vi "Ecal-Manual-2.vi"(0 "PNA_IN":refnum<visa-resource-name>="TCPIP0::169.254.70.180::inst0::INSTR", 1 "RF_Switch_In":refnum<visa-resource-name>="GPIB0::29::INSTR", 5 "error in":errorcluster, 7 "Channel":i32=1, 8 "RecallFile":string="D:\\State Files\\WAM_PRODUCTION.csa", 9 "Save to File(t)":bool=TRUE, 11 "ByPassRfSwitch(t)":bool) -> (12 "Success?(t)":bool, 14 "VISA Out":refnum<visa-resource-name>="TCPIP0::169.254.70.180::inst0::INSTR", 15 "rfsw_out":refnum<visa-resource-name>, 19 "error out":errorcluster)   [LabVIEW 2018]
doc: "This VBScript program performs a Guided Calibration using Mechanical standards. While this example is good to use as a starting point for guided mechanical cal, the Guided comprehensive cal example has some advanced features that are not in this program.\n\nThe SCPI commands in this example are sent over a COM interface using the SCPIStringParser object. You do NOT need a GPIB connection to run this example.\n\nThis VBScript (*.vbs) program can be run as a macro in the PNA. To do this, copy the following code into a text editor file such as Notepad and save it on the PNA hard drive as Guided.vbs. Learn how to setup and run the macro.\n\n' Performing a 2-port cal (Ports 1 and 2)\n\nDim app\nDim scpi\n\n' Create / Get the PNA application.\nSet app = CreateObject(\"AgilentPNA835x.Application\")\nSet scpi = app.ScpiStringParser\n\n' Specify the DUT connectors\nscpi.Execute \"sens:corr:coll:guid:conn:port1 \"\"APC 3.5 female\"\" \"\nscpi.Execute \"sens:corr:coll:guid:conn:port2 \"\"APC 3.5 male\"\" \"\n\n' Note: If your PNA has more than 2 ports, you would need to uncomment\n' one or both of these next two lines, to explicitly specify this is\n' just a 2-port cal.\n'scpi.Execute \"sens:corr:coll:guid:conn:port3 \"\"Not used\"\" \"\n'scpi.Execute \"sens:corr:coll:guid:conn:port4 \"\"Not used\"\" \"\nMsgBox \"Connectors defined for Ports 1 and 2\" \n\n' Select the Cal Kit for each port being calibrated.\nscpi.Execute \"sens:corr:coll:guid:ckit:port1 \"\"85052D\"\" \"\nscpi.Execute \"sens:corr:coll:guid:ckit:port2 \"\"85052D\"\" \"\nMsgBox \"Cal kits defined for Ports 1 and 2\"\n\n' Initiate the calibration and query the number of steps\nscpi.Execute \"sens:corr:coll:guid:init\"\nnumSteps = scpi.Execute(\"sens:corr:coll:guid:steps?\")\nMsgBox \"Number of steps is \" + CStr(numSteps)\n\n' Measure the standards\n'The following series of commands shows that standards \n'can be measured in any order. These steps acquire \n'measurement of standards in reverse order.\n'It is easiest to iterate through standards using \n'a For-Next Loop.\nFor i = numSteps To 1\nstep = \"Step \" + CStr(i) + \" of \" + CStr(numSteps)\nstrPrompt = scpi.Execute(\"sens:corr:coll:guid:desc? \" + CStr(i))\nMsgBox strPrompt, vbOKOnly, step\nscpi.Execute \"sens:corr:coll:guid:acq STAN\" + CStr(i)\nNext\n\n' Conclude the calibration\nscpi.Execute \"sens:corr:coll:guid:save\"\nMsgBox \"Cal is done!\""
uses:
  Instance           1 14Saved   ManCal .vi
  Instruments/PNA-X/PNA-X.lvlib
panel:
  in  "FileSave(path)":string="D:\\State Files\\WAM_PRODUCTION.csa"
  in  "Recall from File(t)":bool=TRUE
  in  "PNA#ofPorts":i32(ring)=2 items=["4"=4, "2"=2]
  in  "PORT 4":bool
  in  "PORT 3":bool
  in  "PORT 2":bool
  in  "PORT 1":bool=TRUE
  in  "Orient":bool=TRUE
  # "Select The Addressess of  VNA and Switch"
  # "Use Bypass Switch if there is no \nswitch controller to connect to"
  # "Select The Number of Ports on the VNA"
  # "Select The Ports on the VNA"
  # "Select VNA Visa Addreess"
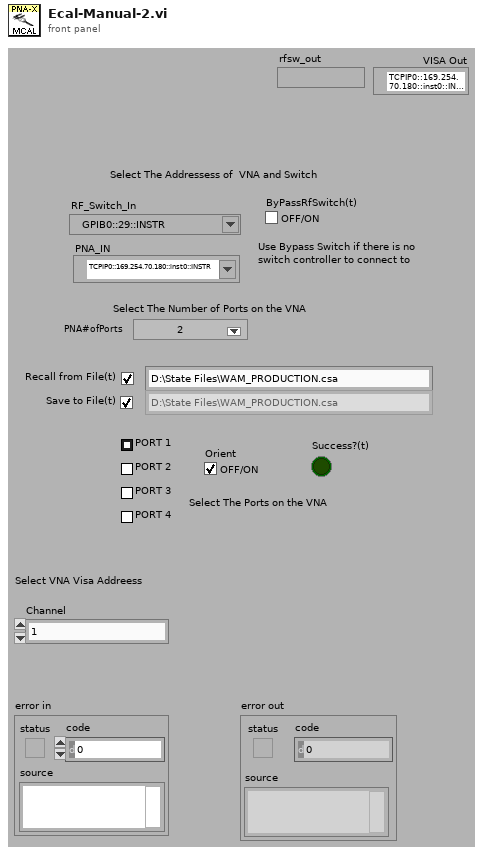
[diagram p1: front panel]
types:
  T1 = enum32{"Invalid", "Standard", "Closed", "Hidden", "Minimized", "Maximized"}
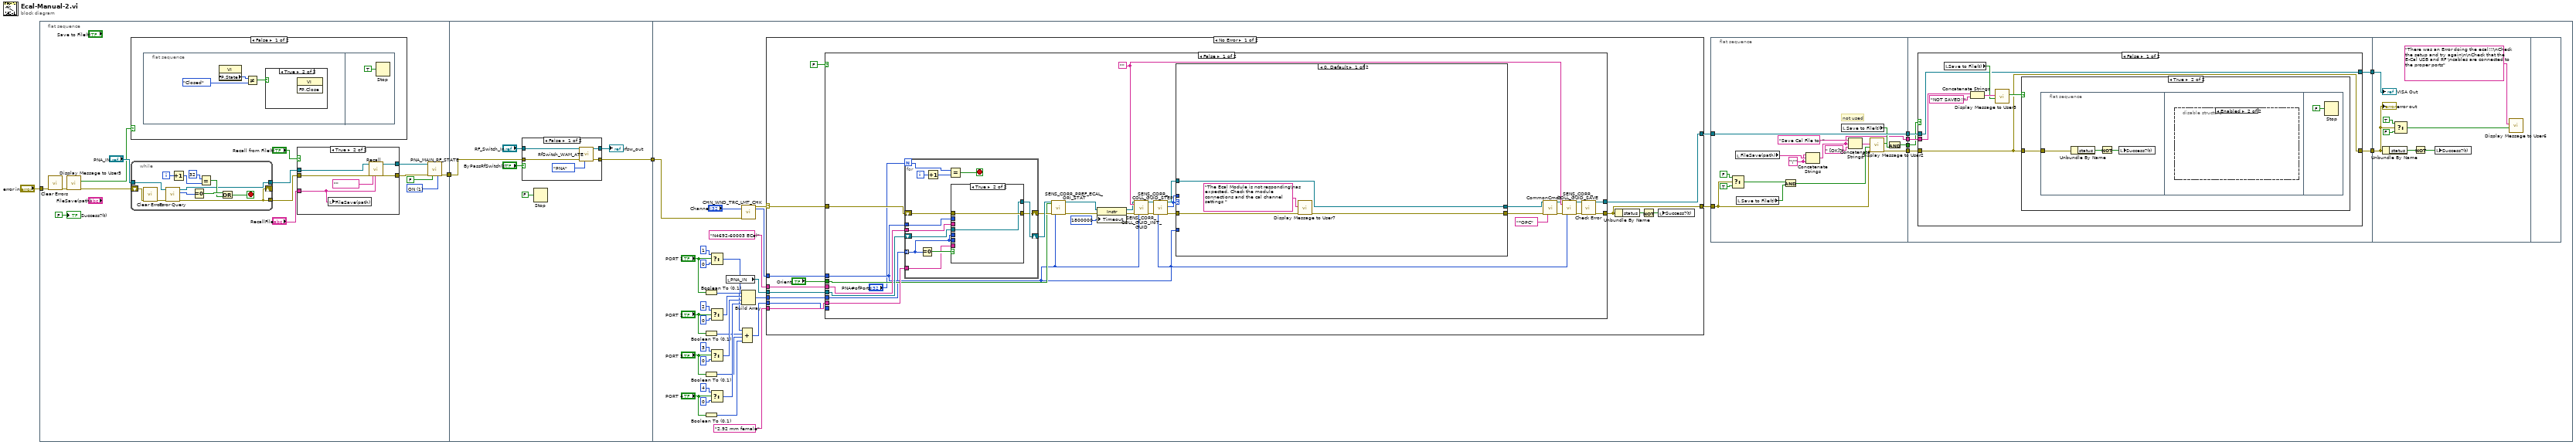
[diagram p0: block diagram]
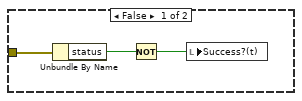
[diagram p6: hidden frame]
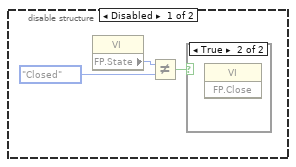
[diagram p7: hidden frame]
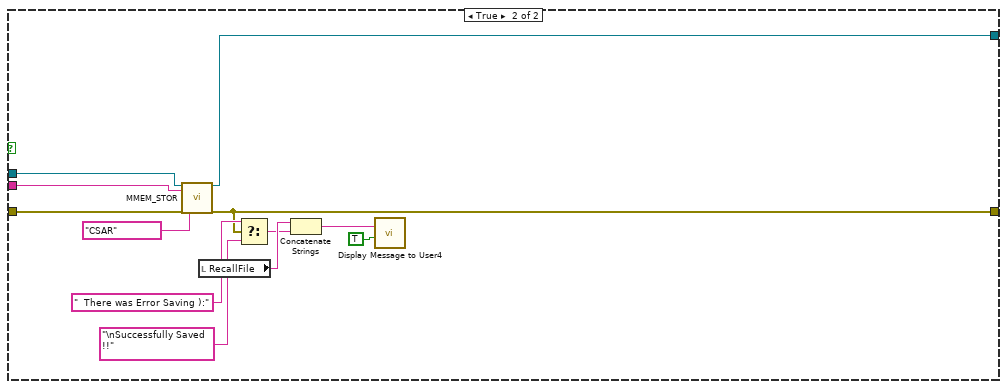
[diagram p9: hidden frame]
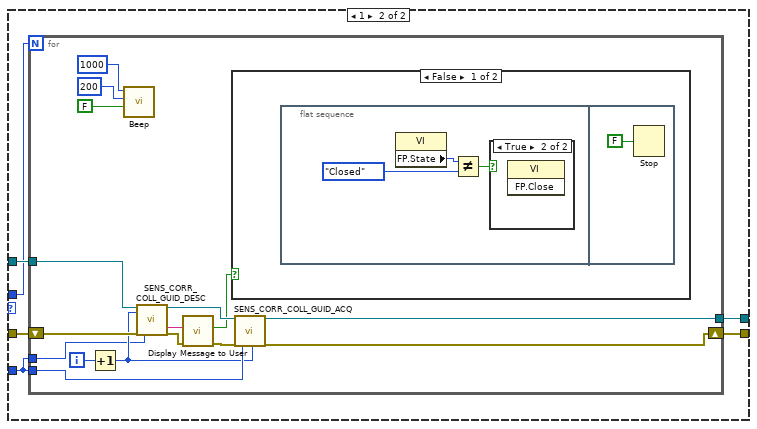
[diagram p10: hidden frame]
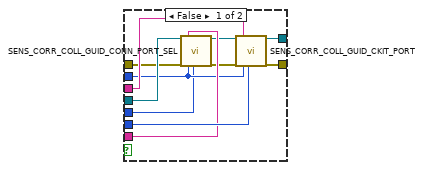
[diagram p13: hidden frame]
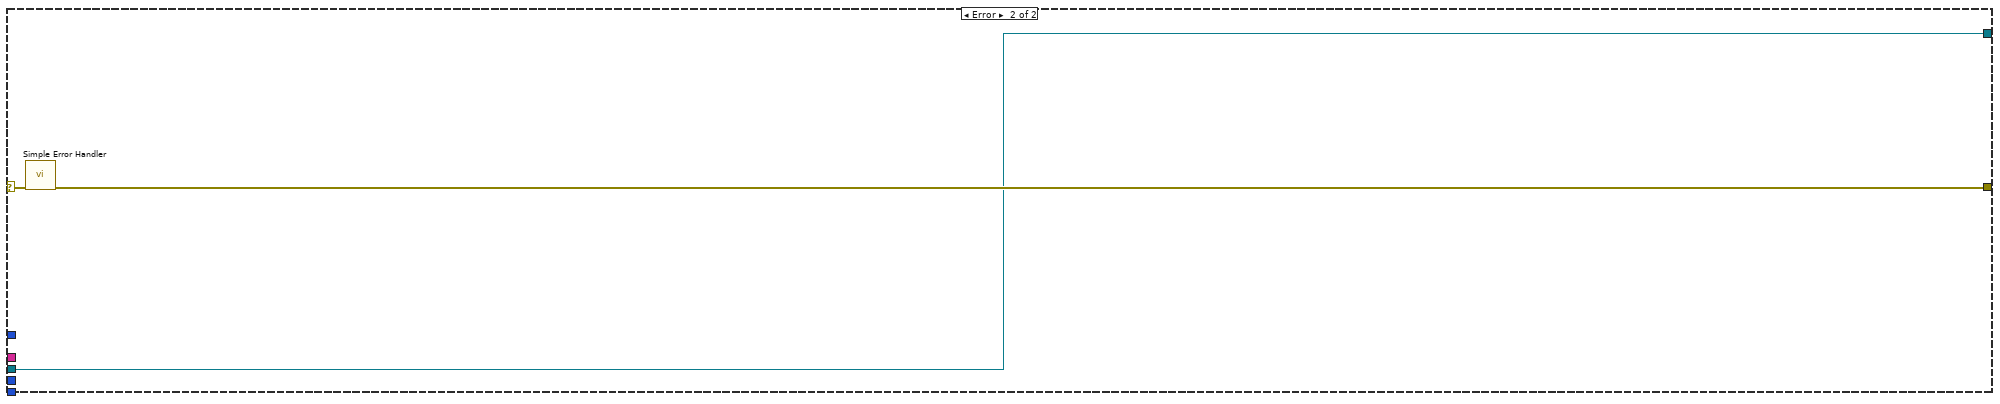
[diagram p15: hidden frame]
diagram:
  n1 = flat-sequence {
    tunnel: "error in" -> [w12]
    tunnel: [w17] -> w1
    tunnel: [w46] -> w3
    tunnel: w1 -> [w47]
    tunnel: w3 -> [w87]
    frame #0 {
      w13 = 1 items=["OFF", "ON"] ("STATE(0=OFF)")
      n2 = call <vilib>:"Clear Errors.vi"("error in (no error)"=w12) -> ("error out"=w11:errorcluster)  [unwired: 5 in, 1 out]
      n3 = call "Display Message to User5"("error in (no error)"=w11) -> ("error out"=w9:errorcluster, "OK"=w5:bool)  [unwired: 9 in]
      n4 = case shown="False" w5 {
        frame False {
          n5 = flat-sequence {
            frame #0 {
              n6 = property class="VI"() -> ("FP.State"=w21:T1)  [unwired: 2 in, 2 out]
              n7 = Not Equal?(x=w21, y=T1."Closed") -> (x != y?=w19:bool)
              n8 = case shown="True" w19 {
                frame False {
                }
                frame True {
                  n9 = invoke class="VI" method="FP.Close"() -> ()  [unwired: 3 in, 3 out]
                }
              }
            }
            frame #1 {
              n10 = Stop(stop? (T)=TRUE) -> ()
            }
          }
        }
        frame True {
        }
      }
      n11 = while {
        shift-right: [w34] -> _
        shift-left: w9 -> [w31]
        tunnel: "PNA_IN" -> [w35]
        tunnel: [w34] -> w8
        tunnel: [w33] -> w7
        i -> [w39]
        stop <- w40 stop-if-true
        n12 = call <vilib>:"Clear Errors.vi"("error in (no error)"=w31) -> ("error out"=w32:errorcluster)  [unwired: 5 in, 1 out]
        n13 = call "Error Query.vi"("error in (no error)"=w32, "VISA Resource Name"=w35) -> ("error out"=w34:errorcluster, "Error"=w41:i32, "dup VISA session"=w33:refnum<visa-resource-name>)  [unwired: 4 in, 1 out]
        n14 = Increment(x=w39) -> (x+1=w36:i32)
        n15 = Equal To 0?(x=w41) -> (x = 0?=w42:bool)
        n16 = Equal?(x=32, y=w36) -> (x = y?=w38:bool)
        n17 = Or(x=w42, y=w38) -> (x .or. y?=w40:bool)
      }
      n18 = case shown="True" "Recall from File(t)" {
        tunnel: "RecallFile" -> [_ w25]
        tunnel: [w23 w30] -> w16
        tunnel: [w24 w29] -> w15
        tunnel: w8 -> [w23 w28]
        tunnel: w7 -> [w24 w27]
        frame False {
        }
        frame True {
          n19 = local write "FileSave(path)"(w25) -> ()
          n20 = call "Recall.vi"("VISA IN"=w27, "error in"=w28, "FileType"="", "FileName"=w25) -> ("VISA Out"=w29:refnum<visa-resource-name>, "error out"=w30:errorcluster)  [unwired: 14 in]
        }
      }
      n21 = call "PNA_MAIN_RF_STATE.vi"("Session In"=w15, "error in"=w16, "RO(T)"=FALSE, "STATE(0=OFF)"=w13) -> ("error out"=w17:errorcluster)  [unwired: 9 in, 2 out]
      "Success?(t)" <- FALSE ("Success?(T)")
    }
    frame #1 {
      n22 = case shown="False" "ByPassRfSwitch(t)" {
        tunnel: "RF_Switch_In" -> [w53 w55]
        tunnel: w47 -> [w52 w54]
        tunnel: [w50 w54] -> w46
        tunnel: [w49 w55] -> w45
        frame False {
          n23 = call "RfSwitch_WAM_ATE.vi"("VISA_IN"=w53, "error in"=w52, "Source"=enum16{"RFSM", "PNA"}."PNA") -> ("visa_out"=w49:refnum<visa-resource-name>, "error out"=w50:errorcluster)  [unwired: 11 in]
        }
        frame True {
        }
      }
      "rfsw_out" <- w45
      n24 = Stop(stop? (T)=FALSE) -> ()
    }
    frame #2 {
      n25 = Boolean To (0,1)(Boolean="PORT 1") -> (0, 1=w72:i16)
      n26 = Boolean To (0,1)(Boolean="PORT 2") -> (0, 1=w73:i16)
      n27 = Boolean To (0,1)(Boolean="PORT 3") -> (0, 1=w74:i16)
      n28 = Boolean To (0,1)(Boolean="PORT 4") -> (0, 1=w75:i16)
      n29 = Select(t=1, s="PORT 1", f=0) -> (s? t:f=w80:i32)
      n30 = Select(t=2, s="PORT 2", f=0) -> (s? t:f=w81:i32)
      n31 = Select(t=3, s="PORT 3", f=0) -> (s? t:f=w82:i32)
      n32 = Select(t=4, s="PORT 4", f=0) -> (s? t:f=w83:i32)
      n33 = local read "PNA_IN"() -> (w84:refnum<visa-resource-name>)
      n34 = call "CHN_WND_TRC_LMT_CHK.vi"("Channel"="Channel", "error in"=w87) -> ("error out"=w88:errorcluster, "Channel"=w89:i32)  [unwired: 13 in, 3 out]
      n35 = Build Array(w80, w81, w82, w83) -> (w86:i32[])
      n36 = Compound Arithmetic op=ADD(w72, w73, w74, w75) -> (w85:i16)
      n37 = case shown="No Error" w88 {
        selector: w88 -> [w163 w256]
        tunnel: [w154 w257] -> w57
        tunnel: w89 -> [w166 _]
        tunnel: w84 -> [w162 w255]
        tunnel: "2.92 mm female" ("Conn") -> [w161 _]
        tunnel: "N4692-60003 ECal" ("CalKit") -> [w160 _]
        tunnel: [w159 w255] -> w61
        tunnel: w85 -> [w158 _]
        tunnel: w86 -> [w157 _]
        frame No Error {
          n38 = case shown="False" FALSE {
            tunnel: [w190 w254] -> w154
            tunnel: w163 -> [w186 w254]
            tunnel: w162 -> [w185 w253]
            tunnel: w160 -> [w184 _]
            tunnel: w161 -> [w183 _]
            tunnel: "Orient" -> [w182 _]
            tunnel: w166 -> [w176 _]
            tunnel: [w175 w253] -> w159
            tunnel: w158 -> [_ _]
            tunnel: w157 -> [w169 _]
            frame False {
              w189 = ""
              n39 = for {
                N: "PNA#ofPorts" -> [w234]
                tunnel: w184 -> [w237]
                tunnel: w183 -> [w228]
                tunnel: w176 -> [w236]
                shift-right: [w238] -> w187
                shift-left: w186 -> [w229]
                shift-right: [w239] -> w188
                shift-left: w185 -> [w230]
                tunnel: w169 -> [w227] mode=indexing
                i -> [w233]
                stop <- w235 stop-if-true
                n40 = Equal To 0?(x=w227) -> (x = 0?=w231:bool)
                n41 = Increment(x=w233) -> (x+1=w232:i32)
                n42 = Equal?(x=w234, y=w232) -> (x = y?=w235:bool)
                n43 = case shown="True" w231 {
                  tunnel: [w250 w252] -> w238
                  tunnel: [w249 w251] -> w239
                  tunnel: w237 -> [w248 _]
                  tunnel: w236 -> [w243 _]
                  tunnel: w227 -> [w247 _]
                  tunnel: w230 -> [w246 w251]
                  tunnel: w229 -> [w245 w252]
                  tunnel: w228 -> [w244 _]
                  tunnel: w227 -> [w242 _]
                  frame False {
                    n44 = call "SENS_CORR_COLL_GUID_CONN_PORT_SEL.vi"("VISA IN"=w246, "error in"=w245, "Port Type"=w244, "Channel"=w243, "Port"=w242) -> ("VISA Out"=w241:refnum<visa-resource-name>, "error out"=w240:errorcluster)  [unwired: 13 in]
                    n45 = call "SENS_CORR_COLL_GUID_CKIT_PORT.vi"("VISA IN"=w241, "error in"=w240, "Ecal ID"=w248, "Channel"=w243, "Port"=w247) -> ("VISA Out"=w249:refnum<visa-resource-name>, "error out"=w250:errorcluster)  [unwired: 13 in]
                  }
                  frame True {
                  }
                }
              }
              n46 = call "SENS_CORR_PREF_ECAL_ORI_STAT.vi"("VISA IN"=w188, "On/Off"=w182, "error in"=w187, "Channel"=w176) -> ("VISA Out"=w181:refnum<visa-resource-name>, "error out"=w178:errorcluster)  [unwired: 14 in]
              n47 = property class="Instr"(reference=w181, error in=w178, "Timeout"=u32 1800000 ("General Settings:Timeout Value")) -> (reference out=w180:refnum<visa-resource-name>, error out=w179:errorcluster)
              n48 = call "SENS_CORR_COLL_GUID_INIT_GUID.vi"("VISA IN"=w180, "Calset"=w189, "error in"=w179, "Channel"=w176) -> ("VISA Out"=w195:refnum<visa-resource-name>, "error out"=w196:errorcluster)  [unwired: 14 in]
              n49 = call "SENS_CORR_COLL_GUID_STEP.vi"("VISA IN"=w195, "error in"=w196, "Channel"=w176) -> ("VISA Out"=w193:refnum<visa-resource-name>, "Data"=w167:i32, "error out"=w194:errorcluster)  [unwired: 14 in]
              n50 = case shown="0, Default" w167 {
                tunnel: w194 -> [w199 w206]
                tunnel: w193 -> [w198 w205]
                tunnel: w167 -> [_ w204]
                tunnel: w176 -> [_ w203]
                tunnel: [w200 w202] -> w173
                tunnel: [w198 w201] -> w172
                frame 0, Default {
                  n51 = call "Display Message to User7"("error in (no error)"=w199, "Message"="The Ecal Module is not responding\nas expected. Check the module connections and the cal channel settings ") -> ("error out"=w200:errorcluster)  [unwired: 8 in, 1 out]
                }
                frame 1 {
                  n52 = for {
                    N: w204 -> [_]
                    tunnel: w205 -> [w220]
                    tunnel: w203 -> [w221]
                    shift-right: [w215] -> w202
                    shift-left: w206 -> [w219]
                    tunnel: [w214] -> w201
                    tunnel: w203 -> [w217]
                    i -> [w222]
                    n53 = Increment(x=w222) -> (x+1=w218:i32)
                    n54 = call <vilib>:"Beep.vi"("use system alert? (T)"=FALSE, "duration (msec)"=u32 200, "frequency (Hz)"=u32 1000) -> ()  [unwired: 9 in]
                    n55 = call "SENS_CORR_COLL_GUID_DESC.vi"("VISA IN"=w220, "Index"=w218, "error in"=w219, "Channel"=w217) -> ("VISA Out"=w216:refnum<visa-resource-name>, "Description"=w211:string, "error out"=w213:errorcluster)  [unwired: 13 in]
                    n56 = call "Display Message to User"("error in (no error)"=w213, "Message"=w211) -> ("error out"=w212:errorcluster, "OK[CONT to CAL}"=w207:bool)  [unwired: 8 in]
                    n57 = case shown="False" w207 {
                      frame False {
                        n58 = flat-sequence {
                          frame #0 {
                            n59 = property class="VI"() -> ("FP.State"=w225:T1)  [unwired: 2 in, 2 out]
                            n60 = Not Equal?(x=w225, y=T1."Closed") -> (x != y?=w223:bool)
                            n61 = case shown="True" w223 {
                              frame False {
                              }
                              frame True {
                                n62 = invoke class="VI" method="FP.Close"() -> ()  [unwired: 3 in, 3 out]
                              }
                            }
                          }
                          frame #1 {
                            n63 = Stop(stop? (T)=FALSE) -> ()
                          }
                        }
                      }
                      frame True {
                      }
                    }
                    n64 = call "SENS_CORR_COLL_GUID_ACQ.vi"("VISA IN"=w216, "error in"=w212, "Channel"=w221, "Standerd"=w218) -> ("VISA Out"=w214:refnum<visa-resource-name>, "error out"=w215:errorcluster)  [unwired: 14 in]
                  }
                }
              }
              n65 = call "CommonCmds.vi"("VISA IN"=w172, "error in"=w173, "Cmds"="*OPC") -> ("VISA Out"=w171:refnum<visa-resource-name>, "error out"=w174:errorcluster)  [unwired: 14 in, 1 out]
              n66 = call "SENS_CORR_COLL_GUID_SAVE.vi"("VISA IN"=w171, "Calset"=w189, "error in"=w174, "Channel"=w176) -> ("VISA Out"=w191:refnum<visa-resource-name>, "error out"=w192:errorcluster)  [unwired: 14 in]
              n67 = call "Check Error.vi"("VISA Resource Name"=w191, "error in (no error)"=w192) -> ("dup VISA session"=w175:refnum<visa-resource-name>, "error out"=w190:errorcluster)  [unwired: 16 in]
            }
            frame True {
            }
          }
          n68 = Unbundle By Name(w154) -> ("status"=w156:bool)
          n69 = Not(x=w156) -> (.not. x?=w155:bool)
          n70 = local write "Success?(t)"(w155) -> ()
        }
        frame Error {
          n71 = call <vilib>:"Simple Error Handler.vi"("error in (no error)"=w256) -> ("error out"=w257:errorcluster)  [unwired: 4 in, 4 out]
        }
      }
      n72 = flat-sequence {
        tunnel: w61 -> [w109]
        tunnel: [w96] -> w60
        tunnel: [w109] -> w59
        tunnel: [w103] -> w58
        tunnel: w57 -> [w104]
        tunnel: [w93] -> w56
        tunnel: [w112] -> w63
        tunnel: [w111] -> w62
        tunnel: w60 -> [w115]
        tunnel: w59 -> [w114]
        tunnel: w58 -> [w113]
        tunnel: w56 -> [w110]
        tunnel: w63 -> [w148]
        tunnel: w62 -> [w149]
        frame #0 {
          w100 = "\"" ("string")
          # "not used"
          n73 = Select(t=FALSE, s=w104, f=TRUE) -> (s? t:f=w107:bool)
          n74 = local read "FileSave(path)"() -> (w102:string)
          n75 = local read "Save to File(t)"() -> (w95:bool)
          n76 = And(x=w107, y=w95) -> (x .and. y?=w108:bool)
          n77 = Concatenate Strings(w100, w102, w100) -> (w96:string)
          n78 = local read "Save to File(t)"() -> (w101:bool)
          n79 = Concatenate Strings("Save Cal File to: " ("Message"), w96, " [OK]?" ("string")) -> (w94:string)
          n80 = call "Display Message to User2"("error in (no error)"=w104, "Enable"=w108, "Message"=w94) -> ("error out"=w103:errorcluster, "OK"=w99:bool)  [unwired: 7 in]
          n81 = And(x=w99, y=w101) -> (x .and. y?=w93:bool)
        }
        frame #1 {
          n82 = case shown="False" w110 {
            tunnel: w115 -> [w122 w145]
            tunnel: w114 -> [w118 w143]
            tunnel: [w116 w135] -> w112
            tunnel: w113 -> [w116 w142]
            tunnel: [w118 w134] -> w111
            frame False {
              n83 = local read "Save to File(t)"() -> (w119:bool)
              n84 = Concatenate Strings(w122, "NOT SAVED!!" ("string")) -> (w121:string)
              n85 = call "Display Message to User3"("Enable"=w119, "Message"=w121) -> ("OK"=w117:bool)  [unwired: 8 in, 1 out]
              n86 = case shown="True" w117 {
                tunnel: w116 -> [w123 w126]
                frame False {
                  n87 = Unbundle By Name(w123) -> ("status"=w124:bool)
                  n88 = Not(x=w124) -> (.not. x?=w125:bool)
                  n89 = local write "Success?(t)"(w125) -> ()
                }
                frame True {
                  n90 = flat-sequence {
                    tunnel: w126 -> [w127]
                    frame #0 {
                      n91 = Unbundle By Name(w127) -> ("status"=w129:bool)
                      n92 = Not(x=w129) -> (.not. x?=w128:bool)
                      n93 = local write "Success?(t)"(w128) -> ()
                    }
                    frame #1 {
                      n94 = disable-structure shown="Enabled" {
                        frame Disabled {
                          n95 = property class="VI"() -> ("FP.State"=w132:T1)  [unwired: 2 in, 2 out]
                          n96 = Not Equal?(x=w132, y=T1."Closed") -> (x != y?=w130:bool)
                          n97 = case shown="True" w130 {
                            frame False {
                            }
                            frame True {
                              n98 = invoke class="VI" method="FP.Close"() -> ()  [unwired: 3 in, 3 out]
                            }
                          }
                        }
                        frame Enabled {
                        }
                      }
                    }
                    frame #2 {
                      n99 = Stop(stop? (T)=FALSE) -> ()
                    }
                  }
                }
              }
            }
            frame True {
              n100 = call "MMEM_STOR.vi"("VISA IN"=w143, "File"=w145, "error in"=w142, "Type"="CSAR") -> ("VISA Out"=w134:refnum<visa-resource-name>, "error out"=w135:errorcluster)  [unwired: 14 in]
              n101 = local read "RecallFile"() -> (w141:string)
              n102 = Select(t="  There was Error Saving ):" ("string"), s=w135, f="\nSuccessfully Saved !!" ("string")) -> (s? t:f=w138:string)
              n103 = Concatenate Strings(w141, w138) -> (w140:string)
              n104 = call "Display Message to User4"("Enable"=TRUE, "Message"=w140) -> ()  [unwired: 8 in, 2 out]
            }
          }
        }
        frame #2 {
          n105 = Unbundle By Name(w148) -> ("status"=w147:bool)
          n106 = Select(t=TRUE, s=w148, f=FALSE) -> (s? t:f=w153:bool)
          n107 = Not(x=w147) -> (.not. x?=w146:bool)
          n108 = local write "Success?(t)"(w146) -> ()
          n109 = call "Display Message to User6"("Enable"=w153, "Message"="There was an Error doing the ecal!!!\nCheck the setup and try again\n\nCheck that the E-Cal USB and RF \ncables are connected to the proper ports") -> ()  [unwired: 8 in, 2 out]
          "error out" <- w148
          "VISA Out" <- w149
        }
        frame #3 {
        }
      }
    }
  }
